vi "Write id info.vi"(8 "error in (no error)":errorcluster, 10 "id info":T1, 11 "Request in":refnum<class "Request.lvclass">) -> (0 "error out":errorcluster, 3 "Request out":refnum<class "Request.lvclass">)   [LabVIEW 2015]
uses:
  Request.lvclass
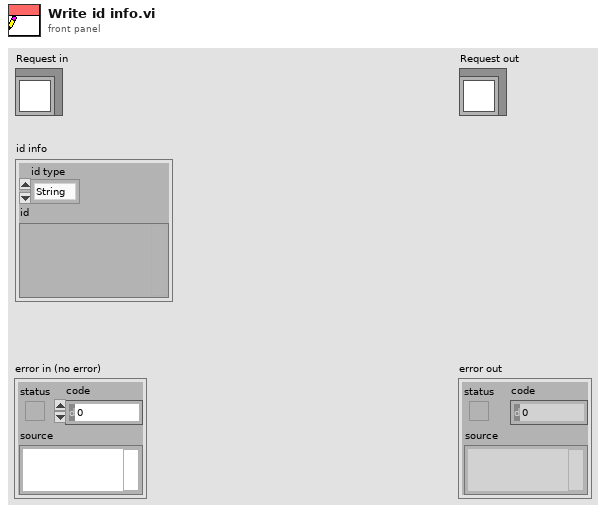
[diagram p1: front panel]
types:
  T1 = cluster{"id type":enum16{"String", "Number", "NULL"}, "id":variant}
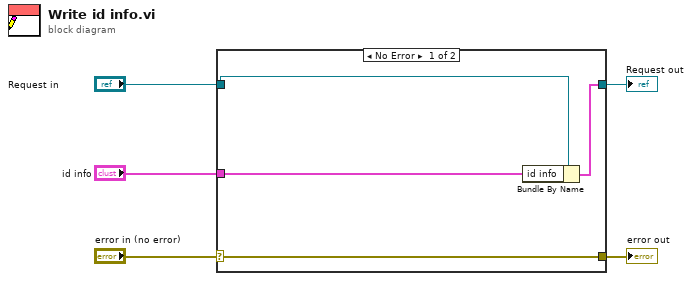
[diagram p0: block diagram]
diagram:
  n1 = case shown="No Error" "error in (no error)" {
    selector: "error in (no error)" -> [w9 w10]
    tunnel: [w9 w10] -> w4
    tunnel: [w7 w11] -> w2
    tunnel: "Request in" -> [w8 w11]
    tunnel: "id info" -> [w6 _]
    frame No Error {
      n2 = Bundle By Name(cluster=w8, "id info"=w6) -> (w7:cluster{})
    }
    frame Error {
    }
  }
  "error out" <- w4
  "Request out" <- w2
